vi "Axsun control.vi"() -> ()   [LabVIEW 2018]
uses:
  General/Controls/QueueNames.ctl
  General/Controls/Queue Manager Actions.ctl
  General/Controls/MessagePacket.ctl
  C:/Project/SerialSectOCT/Software/Axsun/AxsunOCTControlExampleSourceCode_LabVIEW/AxsunOCTControl.dll
  Project/SerialSectOCT/Software/Axsun/AxsunOCTControlExampleSourceCode_LabVIEW/AxsunOCTControl.dll
panel:
  out "Cluster":cluster{i32, string[], string, dbl, string, i32}
  out "GUI error":errorcluster
  in  "Source current OFF":bool
  in  "Source current ON":bool
  in  "stop":bool
  in  "Laser OFF":bool
  in  "Laser ON":bool
  out "processor error":errorcluster
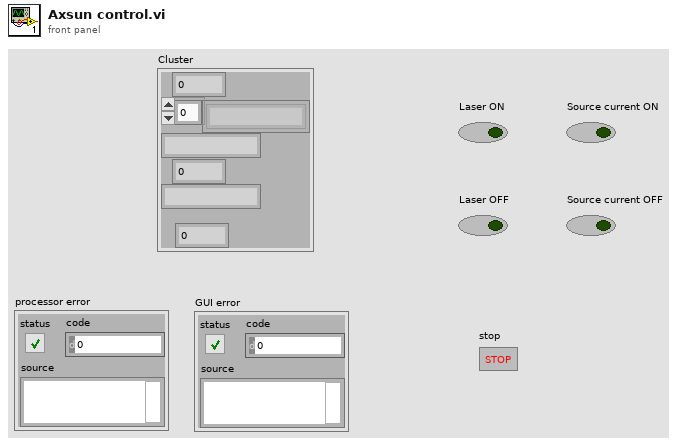
[diagram p1: front panel]
types:
  T1 = typedef "MessagePacket.ctl" = cluster{"Message":string, "Parameter":variant}
  T2 = typedef "Queue Manager Actions.ctl" = enum16{"Init", "Enqueue", "Enqueue All", "Preview Queue", "Dequeue", "Get Status", "Flush Queue", "Flush All Queues", "Release All Queues", "Release Queue", "Enqueue at Opposite End"}
  T3 = typedef "QueueNames.ctl" = enum16{"Main GUI", "Main Scan Processor", "Axsun GUI", "Axsun processor", "Main Display", "Main Table Stage GUI", "Main Table Stage Proc.", "Scan Engine", "Vibratome GUI", "Vibratome Processor", "Slice Engine"}
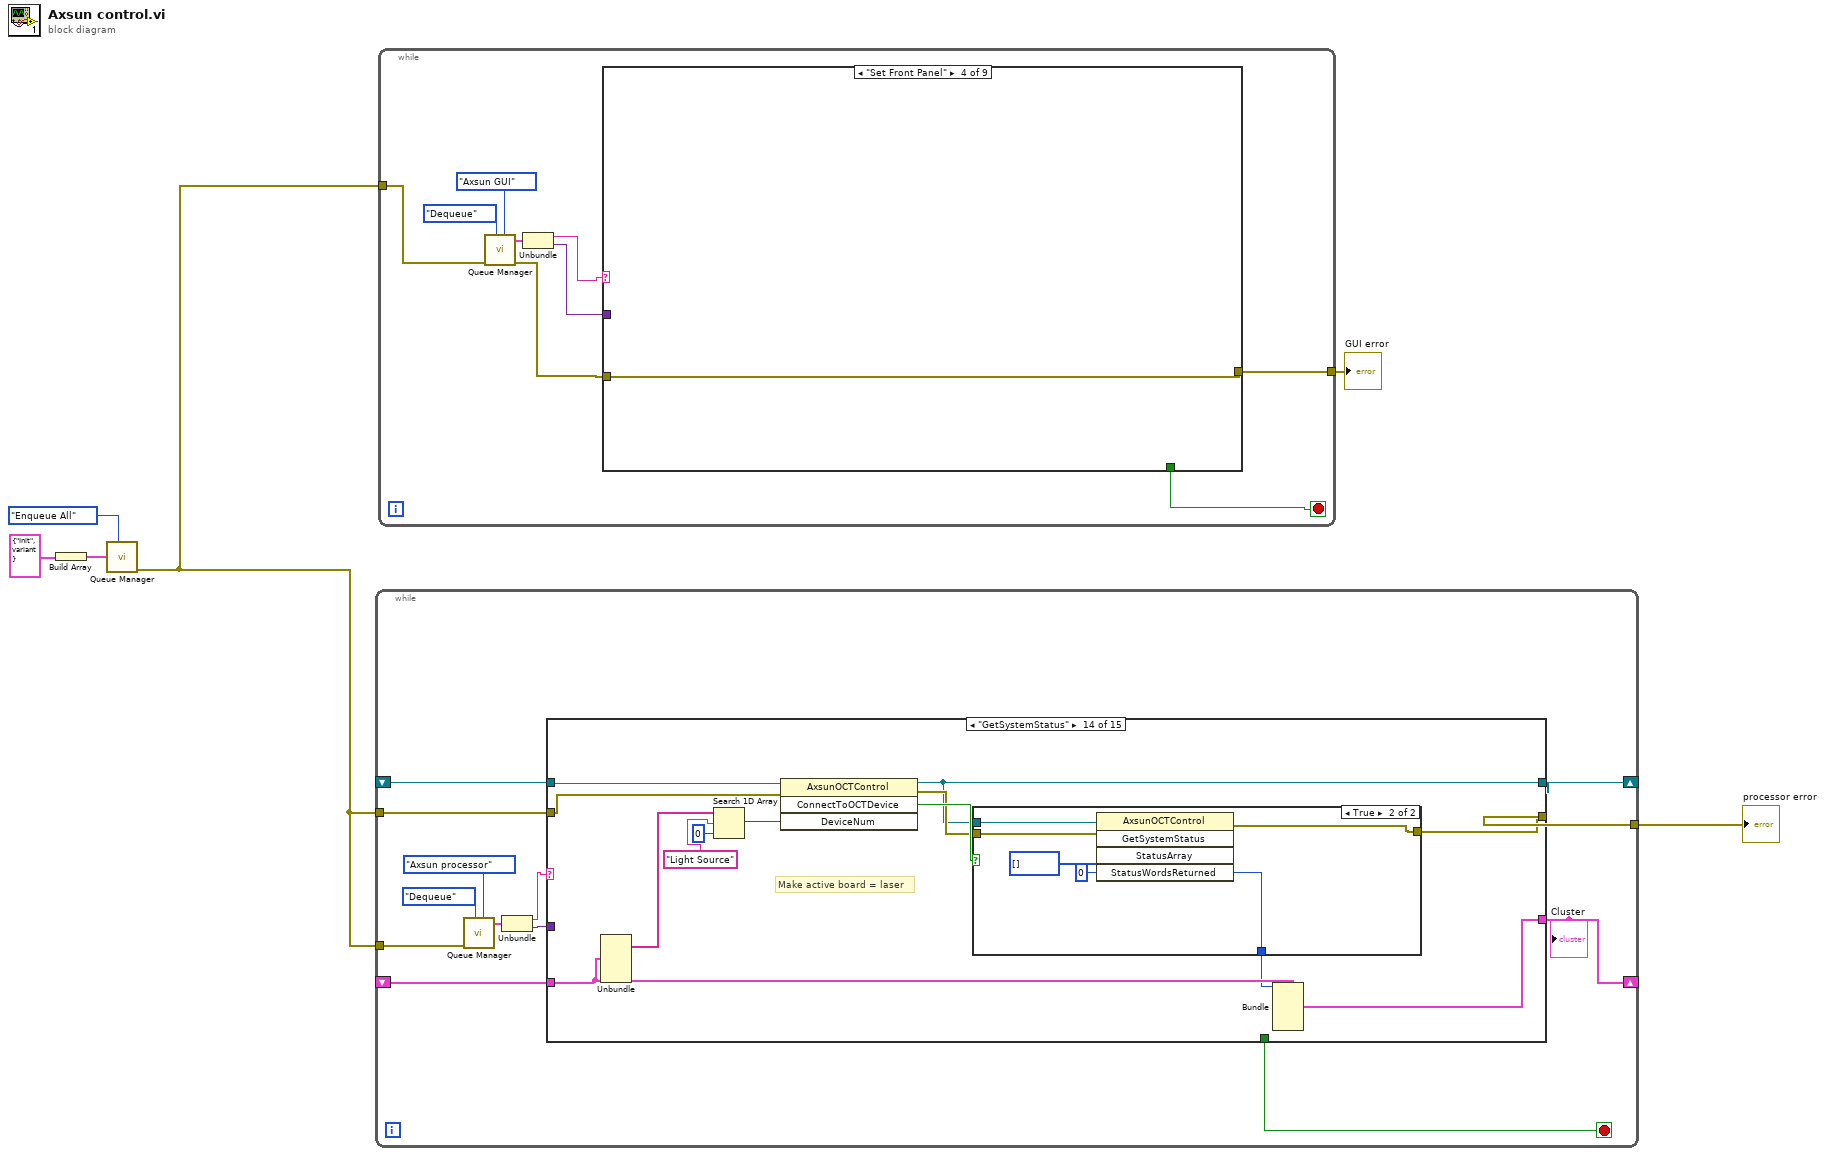
[diagram p0: block diagram]
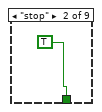
[diagram p3: hidden frame]
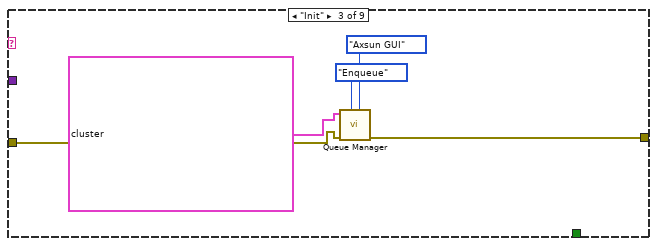
[diagram p4: hidden frame]
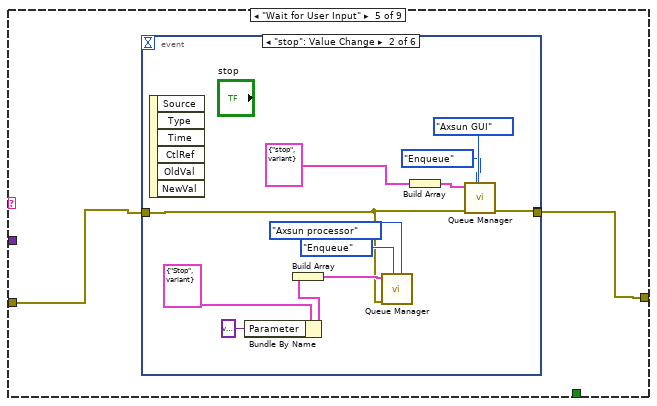
[diagram p5: hidden frame]
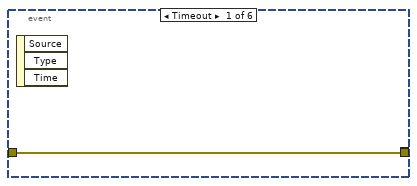
[diagram p6: hidden frame]
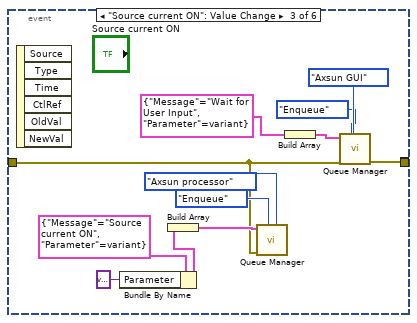
[diagram p7: hidden frame]
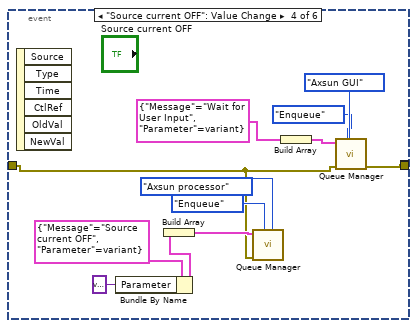
[diagram p8: hidden frame]
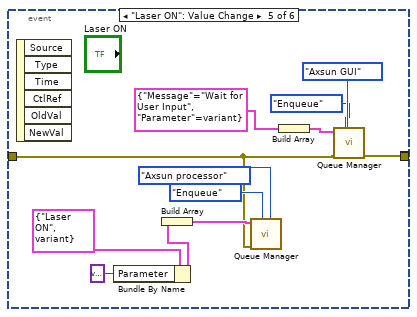
[diagram p9: hidden frame]
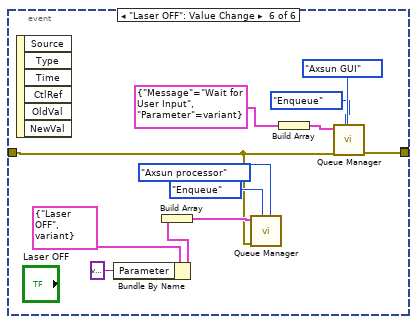
[diagram p10: hidden frame]
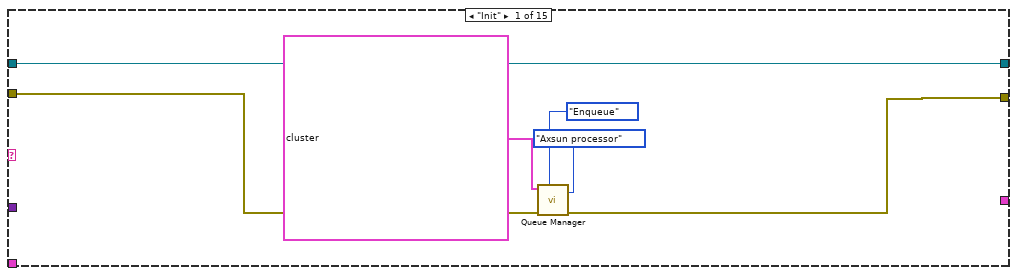
[diagram p15: hidden frame]
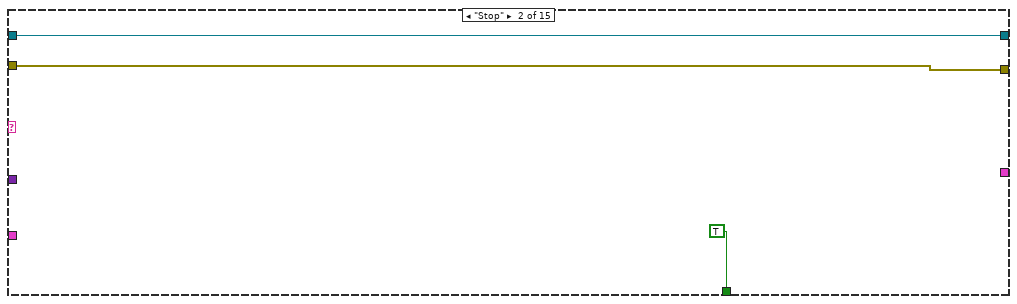
[diagram p16: hidden frame]
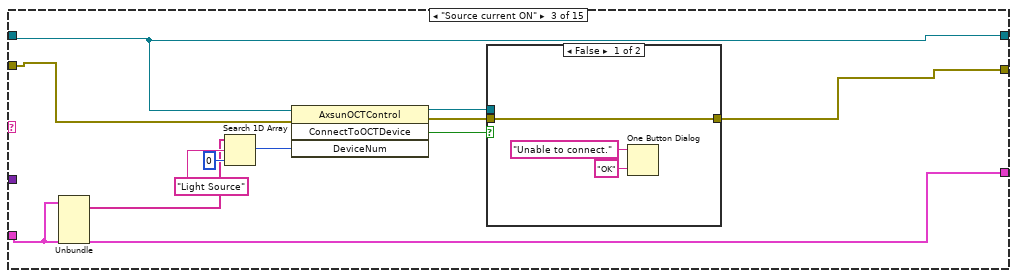
[diagram p17: hidden frame]
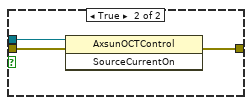
[diagram p18: hidden frame]
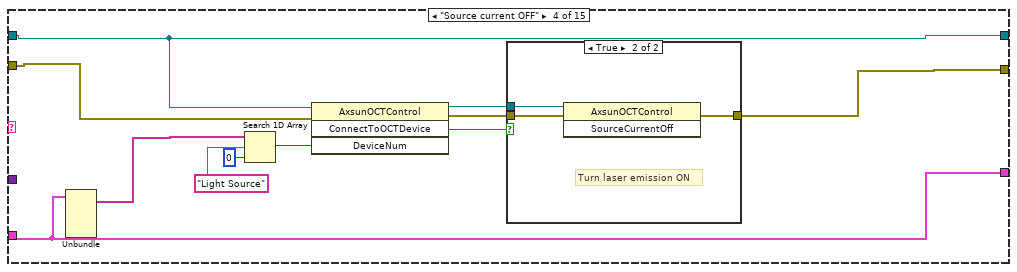
[diagram p19: hidden frame]
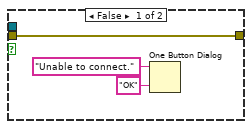
[diagram p20: hidden frame]
diagram:
  n1 = Build Array(T1 {"Message"="Init", "Parameter"=variant} ("Message Packet [In]")) -> (w4:T1[])
  n2 = call "Queue Manager.vi"("Action"=Queue_Manager_Actions."Enqueue All", "Message Packet Array"=w4) -> ("Error Out"=w2:errorcluster)  [unwired: 5 in, 4 out]
  n3 = while {
    shift-right: [w7] -> _
    shift-left: _ -> [w13]
    tunnel: w2 -> [w15]
    shift-right: [w8] -> _
    shift-left: _ -> [w11]
    tunnel: [w10] -> w3
    tunnel: w2 -> [w9]
    stop <- w14 stop-if-true
    n4 = call "Queue Manager.vi"("Queue Name"=QueueNames."Axsun processor", "Action"=Queue_Manager_Actions."Dequeue", "Error In"=w9) -> ("Message Packet [Out]"=w17:T1)  [unwired: 4 in, 4 out]
    n5 = Unbundle(w17) -> ("Message"=w12:string, "Parameter"=w16:variant)
    n6 = case shown="\"GetSystemStatus\"" w12 {
      tunnel: w16 -> [_ _ _ _ _ _ _ _ _ _ _ _ _ _ _]
      tunnel: w15 -> [w25 w27 w33 w49 w65 w70 w86 w106 w124 w146 w165 w183 w190 w212 _]
      tunnel: [_ TRUE _ _ _ _ _ _ _ _ _ _ _ _ _] -> w14
      tunnel: w13 -> [w20 w26 w31 w48 w64 w71 w81 w104 w125 w144 w163 w184 w191 w213 _]
      tunnel: [w21 w27 w32 w50 w65 w68 w82 w105 w123 w145 w164 w182 w185 w207 w229] -> w10
      tunnel: [_ _ w30 w47 w63 w66 w79 w103 w121 w141 w162 w179 w186 w208 w228] -> w8
      tunnel: w11 -> [_ _ w30 w47 w63 w66 _ w103 w122 w143 w162 w180 w188 w210 w228]
      tunnel: [w20 w26 w31 w48 w64 w67 w81 w104 w125 w144 w163 w181 w191 w206 w230] -> w7
      frame "Init" {
        n7 = call "Queue Manager.vi"("Queue Name"=QueueNames."Axsun processor", "Action"=Queue_Manager_Actions."Enqueue", "Error In"=w25, "Message Packet Array"=T1[] [{"Message"="Create handle", "Parameter"=variant}, {"Message"="Start Network Control Interface", "Parameter"=variant}, {"Message"="Get laser handle", "Parameter"=variant}, {"Message"="GetControlVersion", "Parameter"=variant}, {"Message"="GetSerialNum", "Parameter"=variant}, {"Message"="GetSystemStatus", "Parameter"=variant}, {"Message"="GetWaveLengthAtSweptTrigger", "Parameter"=variant}, {"Message"="GetLaserOnTime\nGetLaserOnTime", "Parameter"=variant}]) -> ("Error Out"=w21:errorcluster)  [unwired: 3 in, 4 out]
      }
      frame "Stop" {
      }
      frame "Source current ON" {
        n8 = Unbundle(w30) -> (w29:string[])  [unwired: 5 out]
        n9 = Search 1D Array(1D array=w29, element="Light Source", start index (0)=0) -> (index of element=w37:i32)
        n10 = invoke class="AxsunOCTControl" method="ConnectToOCTDevice"(reference=w31, error in=w33, "DeviceNum"=w37) -> (reference out=w36:refnum<k24>, error out=w35:errorcluster, "ConnectToOCTDevice"=w34:bool)  [unwired: 1 in, 1 out]
        n11 = case shown="False" w34 {
          tunnel: w36 -> [_ w45]
          tunnel: w35 -> [w42 w44]
          tunnel: [w42 w43] -> w32
          frame False {
            n12 = One Button Dialog(message="Unable to connect.", button name ("OK")="OK") -> ()  [unwired: 1 out]
          }
          frame True {
            n13 = invoke class="AxsunOCTControl" method="SourceCurrentOn"(reference=w45, error in=w44) -> (error out=w43:errorcluster)  [unwired: 1 in, 2 out]
          }
        }
      }
      frame "Source current OFF" {
        n14 = Unbundle(w47) -> (w46:string[])  [unwired: 5 out]
        n15 = Search 1D Array(1D array=w46, element="Light Source", start index (0)=0) -> (index of element=w54:i32)
        n16 = invoke class="AxsunOCTControl" method="ConnectToOCTDevice"(reference=w48, error in=w49, "DeviceNum"=w54) -> (reference out=w53:refnum<k24>, error out=w52:errorcluster, "ConnectToOCTDevice"=w51:bool)  [unwired: 1 in, 1 out]
        n17 = case shown="True" w51 {
          tunnel: w53 -> [_ w62]
          tunnel: w52 -> [w59 w61]
          tunnel: [w59 w60] -> w50
          frame False {
            n18 = One Button Dialog(message="Unable to connect.", button name ("OK")="OK") -> ()  [unwired: 1 out]
          }
          frame True {
            # "Turn laser emission ON"
            n19 = invoke class="AxsunOCTControl" method="SourceCurrentOff"(reference=w62, error in=w61) -> (error out=w60:errorcluster)  [unwired: 1 in, 2 out]
          }
        }
      }
      frame Default {
      }
      frame "Start Network Control Interface" {
        n20 = invoke class="AxsunOCTControl" method="StartNetworkControlInterface"(reference=w71, error in=w70) -> (reference out=w67:refnum<k24>, error out=w69:errorcluster)  [unwired: 1 in, 1 out]
        n21 = flat-sequence {
          tunnel: w69 -> [w72]
          tunnel: [w72] -> w68
          frame #0 {
            n22 = Wait (ms)(milliseconds to wait=2000) -> ()  [unwired: 1 out]
          }
        }
      }
      frame "Get laser handle" {
        n23 = invoke class="AxsunOCTControl" method="GetNumberOfOCTDevicesPresent"(reference=w81, error in=w86) -> (reference out=w85:refnum<k24>, error out=w83:errorcluster, "GetNumberOfOCTDevicesPresent"=w84:i32)  [unwired: 1 in]
        n24 = for {
          N: w84 -> [_]
          tunnel: w85 -> [w92]
          tunnel: w83 -> [w91]
          tunnel: [w87] -> w80 mode=indexing
          tunnel: [w89] -> w82
          tunnel: [w88] -> _ mode=indexing
          i -> [w90]
          n25 = invoke class="AxsunOCTControl" method="ConnectToOCTDevice"(reference=w92, error in=w91, "DeviceNum"=w90) -> (reference out=w96:refnum<k24>, error out=w95:errorcluster)  [unwired: 1 in, 2 out]
          n26 = stacked-sequence {
            tunnel: w96 -> [w101]
            tunnel: [w101] -> w94
            tunnel: w95 -> [w100]
            tunnel: [w100] -> w93
            frame #0 {
              n27 = Wait (ms)(milliseconds to wait=u32 20) -> ()  [unwired: 1 out]
            }
          }
          n28 = invoke class="AxsunOCTControl" method="GetSystemType"(reference=w94, error in=w93, "SystemType"=u32 0, "SystemTypeString"="") -> (reference out=w88:refnum<k24>, error out=w89:errorcluster, "SystemTypeString"=w87:string)  [unwired: 1 in, 2 out]
        }
        n29 = Bundle(0, w80, "GetControlVersion", 0.0, "", 0) -> (w79:cluster{i32, string[], string, dbl, string, i32})  [unwired: 1 in]
      }
      frame "Laser ON" {
        n30 = Unbundle(w103) -> (w102:string[])  [unwired: 5 out]
        n31 = Search 1D Array(1D array=w102, element="Light Source", start index (0)=0) -> (index of element=w110:i32)
        n32 = invoke class="AxsunOCTControl" method="ConnectToOCTDevice"(reference=w104, error in=w106, "DeviceNum"=w110) -> (reference out=w109:refnum<k24>, error out=w108:errorcluster, "ConnectToOCTDevice"=w107:bool)  [unwired: 1 in, 1 out]
        n33 = case shown="True" w107 {
          tunnel: w109 -> [_ w118]
          tunnel: w108 -> [w115 w117]
          tunnel: [w115 w116] -> w105
          frame False {
            n34 = One Button Dialog(message="Unable to .", button name ("OK")="OK") -> ()  [unwired: 1 out]
          }
          frame True {
            # "Turn laser emission ON"
            n35 = invoke class="AxsunOCTControl" method="StartScan"(reference=w118, error in=w117) -> (error out=w116:errorcluster)  [unwired: 1 in, 2 out]
          }
        }
      }
      frame "GetWaveLengthAtSweptTrigger" {
        n36 = Unbundle(w122) -> (w120:string[])  [unwired: 5 out]
        n37 = Search 1D Array(1D array=w120, element="Light Source", start index (0)=0) -> (index of element=w129:i32)
        n38 = invoke class="AxsunOCTControl" method="ConnectToOCTDevice"(reference=w125, error in=w124, "DeviceNum"=w129) -> (reference out=w128:refnum<k24>, error out=w127:errorcluster, "ConnectToOCTDevice"=w126:bool)  [unwired: 1 in, 1 out]
        n39 = case shown="False" w126 {
          tunnel: w128 -> [_ w139]
          tunnel: w127 -> [w134 w138]
          tunnel: [w134 w137] -> w123
          tunnel: [_ w135] -> w119
          frame False {
            n40 = One Button Dialog(message="Unable to .", button name ("OK")="OK") -> ()  [unwired: 1 out]
          }
          frame True {
            # "Turn laser emission ON"
            n41 = invoke class="AxsunOCTControl" method="GetWavelengthAtSweepTrigger"(reference=w139, error in=w138, "Wavelength"=0.0) -> (error out=w137:errorcluster, "Wavelength"=w135:dbl)  [unwired: 1 in, 2 out]
          }
        }
        n42 = Bundle(cluster=w122, w119) -> (w121:cluster{i32, string[], string, dbl, string, i32})  [unwired: 5 in]
      }
      frame "GetLaserOnTime" {
        # "Make active board = laser"
        n43 = Unbundle(w143) -> (w140:string[])  [unwired: 5 out]
        n44 = Search 1D Array(1D array=w140, element="Light Source", start index (0)=0) -> (index of element=w152:i32)
        n45 = invoke class="AxsunOCTControl" method="ConnectToOCTDevice"(reference=w144, error in=w146, "DeviceNum"=w152) -> (reference out=w148:refnum<k24>, error out=w149:errorcluster, "ConnectToOCTDevice"=w147:bool)  [unwired: 1 in, 1 out]
        n46 = case shown="False" w147 {
          tunnel: w149 -> [w155 w159]
          tunnel: w148 -> [_ w160]
          tunnel: [w155 w158] -> w145
          tunnel: [_ w156] -> w142
          frame False {
            n47 = One Button Dialog(message="Unable to connect.", button name ("OK")="OK") -> ()  [unwired: 1 out]
          }
          frame True {
            n48 = invoke class="AxsunOCTControl" method="GetLaserOnTime"(reference=w160, error in=w159, "LaserOnTimeSeconds"=u32 0) -> (error out=w158:errorcluster, "LaserOnTimeSeconds"=w156:u32)  [unwired: 1 in, 2 out]
          }
        }
        n49 = Bundle(cluster=w143, w142) -> (w141:cluster{i32, string[], string, dbl, string, i32})  [unwired: 5 in]
      }
      frame "Laser OFF" {
        # "Make active board = laser"
        n50 = Unbundle(w162) -> (w161:string[])  [unwired: 5 out]
        n51 = Search 1D Array(1D array=w161, element="Light Source", start index (0)=0) -> (index of element=w169:i32)
        n52 = invoke class="AxsunOCTControl" method="ConnectToOCTDevice"(reference=w163, error in=w165, "DeviceNum"=w169) -> (reference out=w168:refnum<k24>, error out=w167:errorcluster, "ConnectToOCTDevice"=w166:bool)  [unwired: 1 in, 1 out]
        n53 = case shown="True" w166 {
          tunnel: w168 -> [_ w177]
          tunnel: w167 -> [w174 w176]
          tunnel: [w174 w175] -> w164
          frame False {
            n54 = One Button Dialog(message="Unable to connect.", button name ("OK")="OK") -> ()  [unwired: 1 out]
          }
          frame True {
            # "Turn laser emission ON"
            n55 = invoke class="AxsunOCTControl" method="StopScan"(reference=w177, error in=w176) -> (error out=w175:errorcluster)  [unwired: 1 in, 2 out]
          }
        }
      }
      frame "GetControlVersion" {
        n56 = invoke class="AxsunOCTControl" method="GetControlVersion"(reference=w184, error in=w183) -> (reference out=w181:refnum<k24>, error out=w182:errorcluster, "GetControlVersion"=w178:string)  [unwired: 1 in]
        n57 = Bundle(cluster=w180, w178) -> (w179:cluster{i32, string[], string, dbl, string, i32})  [unwired: 5 in]
      }
      frame "GetSerialNum" {
        n58 = Unbundle(w188) -> (w189:string[])  [unwired: 5 out]
        n59 = Search 1D Array(1D array=w189, element="Light Source", start index (0)=0) -> (index of element=w195:i32)
        n60 = invoke class="AxsunOCTControl" method="ConnectToOCTDevice"(reference=w191, error in=w190, "DeviceNum"=w195) -> (reference out=w194:refnum<k24>, error out=w193:errorcluster, "ConnectToOCTDevice"=w192:bool)  [unwired: 1 in, 1 out]
        n61 = case shown="True" w192 {
          tunnel: w194 -> [_ w205]
          tunnel: w193 -> [w200 w204]
          tunnel: [w200 w203] -> w185
          tunnel: [_ w201] -> w187
          frame False {
            n62 = One Button Dialog(message="Unable to connect.", button name ("OK")="OK") -> ()  [unwired: 1 out]
          }
          frame True {
            n63 = invoke class="AxsunOCTControl" method="GetSerialNum"(reference=w205, error in=w204, "SerialNum"="") -> (error out=w203:errorcluster, "SerialNum"=w201:string)  [unwired: 1 in, 2 out]
          }
        }
        n64 = Bundle(cluster=w188, w187) -> (w186:cluster{i32, string[], string, dbl, string, i32})  [unwired: 5 in]
      }
      frame "GetSystemStatus" {
        # "Make active board = laser"
        n65 = Unbundle(w210) -> (w211:string[])  [unwired: 5 out]
        n66 = Search 1D Array(1D array=w211, element="Light Source", start index (0)=0) -> (index of element=w218:i32)
        n67 = invoke class="AxsunOCTControl" method="ConnectToOCTDevice"(reference=w213, error in=w212, "DeviceNum"=w218) -> (reference out=w206:refnum<k24>, error out=w214:errorcluster, "ConnectToOCTDevice"=w215:bool)  [unwired: 1 in, 1 out]
        n68 = case shown="True" w215 {
          tunnel: w214 -> [w221 w226]
          tunnel: w206 -> [_ w227]
          tunnel: [w221 w223] -> w207
          tunnel: [_ w222] -> w209
          frame False {
            n69 = One Button Dialog(message="Unable to connect.", button name ("OK")="OK") -> ()  [unwired: 1 out]
          }
          frame True {
            n70 = invoke class="AxsunOCTControl" method="GetSystemStatus"(reference=w227, error in=w226, "StatusArray"=u32[] [], "StatusWordsReturned"=u32 0) -> (error out=w223:errorcluster, "StatusWordsReturned"=w222:u32)  [unwired: 1 in, 3 out]
          }
        }
        n71 = Bundle(cluster=w210, w209) -> (w208:cluster{i32, string[], string, dbl, string, i32})  [unwired: 5 in]
      }
      frame "Create handle" {
        n72 = constructor class="AxsunOCTControl"() -> (reference out=w230:refnum<k24>, error out=w229:errorcluster)  [unwired: 3 in, 1 out]
      }
    }
    "Cluster" <- w8
  }
  "processor error" <- w3
  n73 = while {
    tunnel: w2 -> [w236]
    tunnel: [w232] -> w1
    stop <- w231 stop-if-true
    n74 = call "Queue Manager.vi"("Queue Name"=QueueNames."Axsun GUI", "Action"=Queue_Manager_Actions."Dequeue", "Error In"=w236) -> ("Error Out"=w233:errorcluster, "Message Packet [Out]"=w237:T1)  [unwired: 4 in, 3 out]
    n75 = Unbundle(w237) -> ("Message"=w235:string, "Parameter"=w234:variant)
    n76 = case shown="\"Set Front Panel\"" w235 {
      tunnel: w234 -> [_ _ _ _ _ _ _ _ _]
      tunnel: w233 -> [w240 _ w246 w247 w249 w311 w312 w313 w314]
      tunnel: [w240 _ w243 w247 w248 w311 w312 w313 w314] -> w232
      tunnel: [_ TRUE _ _ _ _ _ _ _] -> w231
      frame "False", Default {
      }
      frame "stop" {
      }
      frame "Init" {
        n77 = call "Queue Manager.vi"("Queue Name"=QueueNames."Axsun GUI", "Action"=Queue_Manager_Actions."Enqueue", "Error In"=w246, "Message Packet Array"=T1[] [{"Message"="Wait for Complete", "Parameter"=variant}, {"Message"="Set Front Panel", "Parameter"=variant}, {"Message"="Load User Settings", "Parameter"=variant}, {"Message"="Configure Hardware", "Parameter"=variant}, {"Message"="Configure Hardware", "Parameter"=variant}, {"Message"="Wait for User Input", "Parameter"=variant}]) -> ("Error Out"=w243:errorcluster)  [unwired: 3 in, 4 out]
      }
      frame "Set Front Panel" {
      }
      frame "Wait for User Input" {
        n78 = event shown="[1] \"stop\": Value Change" {
          selector: _ -> [_ _ _ _ _ _]
          dyn-events: _ -> [_ _ _ _ _ _]
          timeout: _ -> [_ _ _ _ _ _]
          tunnel: w249 -> [w250 w251 w263 w275 w287 w299]
          tunnel: [_ w252 w264 w276 w291 w301] -> w248
          tunnel: [w250 _ _ _ _ _] -> _
          event Timeout {
            n79 = event-data() -> ()  [unwired: 1 in, 3 out]
          }
          event "stop": Value Change {
            n80 = event-data() -> ()  [unwired: 1 in, 6 out]
            n81 = Bundle By Name(cluster=T1 {"Message"="Stop", "Parameter"=variant} ("Message Packet [In]"), "Parameter"=variant) -> (w258:T1)
            n82 = Build Array(w258) -> (w255:T1[])
            n83 = call "Queue Manager.vi"("Queue Name"=QueueNames."Axsun processor", "Action"=Queue_Manager_Actions."Enqueue", "Error In"=w251, "Message Packet Array"=w255) -> ()  [unwired: 3 in, 5 out]
            n84 = Build Array(T1 {"Message"="stop", "Parameter"=variant} ("Message Packet [In]")) -> (w262:T1[])
            n85 = call "Queue Manager.vi"("Queue Name"=QueueNames."Axsun GUI", "Action"=Queue_Manager_Actions."Enqueue", "Error In"=w251, "Message Packet Array"=w262) -> ("Error Out"=w252:errorcluster)  [unwired: 3 in, 4 out]
          }
          event "Source current ON": Value Change {
            n86 = event-data() -> ()  [unwired: 1 in, 6 out]
            n87 = Bundle By Name(cluster=T1 {"Message"="Source current ON", "Parameter"=variant} ("Message Packet [In]"), "Parameter"=variant) -> (w270:T1)
            n88 = Build Array(w270) -> (w267:T1[])
            n89 = call "Queue Manager.vi"("Queue Name"=QueueNames."Axsun processor", "Action"=Queue_Manager_Actions."Enqueue", "Error In"=w263, "Message Packet Array"=w267) -> ()  [unwired: 3 in, 5 out]
            n90 = Build Array(T1 {"Message"="Wait for User Input", "Parameter"=variant} ("Message Packet [In]")) -> (w274:T1[])
            n91 = call "Queue Manager.vi"("Queue Name"=QueueNames."Axsun GUI", "Action"=Queue_Manager_Actions."Enqueue", "Error In"=w263, "Message Packet Array"=w274) -> ("Error Out"=w264:errorcluster)  [unwired: 3 in, 4 out]
          }
          event "Source current OFF": Value Change {
            n92 = event-data() -> ()  [unwired: 1 in, 6 out]
            n93 = Bundle By Name(cluster=T1 {"Message"="Source current OFF", "Parameter"=variant} ("Message Packet [In]"), "Parameter"=variant) -> (w282:T1)
            n94 = Build Array(w282) -> (w279:T1[])
            n95 = call "Queue Manager.vi"("Queue Name"=QueueNames."Axsun processor", "Action"=Queue_Manager_Actions."Enqueue", "Error In"=w275, "Message Packet Array"=w279) -> ()  [unwired: 3 in, 5 out]
            n96 = Build Array(T1 {"Message"="Wait for User Input", "Parameter"=variant} ("Message Packet [In]")) -> (w286:T1[])
            n97 = call "Queue Manager.vi"("Queue Name"=QueueNames."Axsun GUI", "Action"=Queue_Manager_Actions."Enqueue", "Error In"=w275, "Message Packet Array"=w286) -> ("Error Out"=w276:errorcluster)  [unwired: 3 in, 4 out]
          }
          event "Laser ON": Value Change {
            n98 = event-data() -> ()  [unwired: 1 in, 6 out]
            n99 = Bundle By Name(cluster=T1 {"Message"="Laser ON", "Parameter"=variant} ("Message Packet [In]"), "Parameter"=variant) -> (w294:T1)
            n100 = Build Array(w294) -> (w290:T1[])
            n101 = call "Queue Manager.vi"("Queue Name"=QueueNames."Axsun processor", "Action"=Queue_Manager_Actions."Enqueue", "Error In"=w287, "Message Packet Array"=w290) -> ()  [unwired: 3 in, 5 out]
            n102 = Build Array(T1 {"Message"="Wait for User Input", "Parameter"=variant} ("Message Packet [In]")) -> (w298:T1[])
            n103 = call "Queue Manager.vi"("Queue Name"=QueueNames."Axsun GUI", "Action"=Queue_Manager_Actions."Enqueue", "Error In"=w287, "Message Packet Array"=w298) -> ("Error Out"=w291:errorcluster)  [unwired: 3 in, 4 out]
          }
          event "Laser OFF": Value Change {
            n104 = event-data() -> ()  [unwired: 1 in, 6 out]
            n105 = Bundle By Name(cluster=T1 {"Message"="Laser OFF", "Parameter"=variant} ("Message Packet [In]"), "Parameter"=variant) -> (w306:T1)
            n106 = Build Array(w306) -> (w303:T1[])
            n107 = call "Queue Manager.vi"("Queue Name"=QueueNames."Axsun processor", "Action"=Queue_Manager_Actions."Enqueue", "Error In"=w299, "Message Packet Array"=w303) -> ()  [unwired: 3 in, 5 out]
            n108 = Build Array(T1 {"Message"="Wait for User Input", "Parameter"=variant} ("Message Packet [In]")) -> (w310:T1[])
            n109 = call "Queue Manager.vi"("Queue Name"=QueueNames."Axsun GUI", "Action"=Queue_Manager_Actions."Enqueue", "Error In"=w299, "Message Packet Array"=w310) -> ("Error Out"=w301:errorcluster)  [unwired: 3 in, 4 out]
          }
        }
      }
      frame "Wait for Complete" {
      }
      frame "Configure Hardware" {
      }
      frame "Load User Settings" {
      }
      frame "Init Variables" {
      }
    }
  }
  "GUI error" <- w1
